vi "5Pixel.vi"() -> (3 "5 pixel":u32)   [LabVIEW 2009, in "menu item.lvclass"]
uses:
  menu item.lvclass
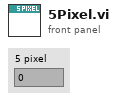
[diagram p1: front panel]
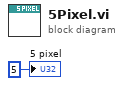
[diagram p0: block diagram]
diagram:
  "5 pixel" <- u32 5 ("1 pixel")
